vi "PSA-Mask.vi"(6 "Freq(GHZ)":dbl=20.0, 7 "Mask Offset dB":dbl, 9 "Error (dBin)":dbl, 11 "Att":dbl=0.5) -> (2 "Array":dbl[](array[numeric])=[0.5, 1.1724999999999999, 0.5862499999999999, -0.5862499999999999, 0.0], 3 "parsed result":string[](array[string]), 5 "Pass(t)":bool)   [LabVIEW 2018]
panel:
  out "Array(str)":string[](array[string])=["0.5", "1.172", "0.586", "-0.586", "0"]
  # "Error In,Atten(db),HSL,LSL,Error(db)-, Error(db)+, p/f"
  # "Error In, Atten(db),Error,Error(db)-, Error(db)+, p/f"
  # "https://ragesystems.sharepoint.com/:b:/r/sites/Tetra/Shared%20Documents/Design%20Docs/Data%20Sheets/Peregrine%20Step%20Atten%206b%2031db%2045G%20PE43614ds.pdf?csf=1&web=1&e=NTfwej"
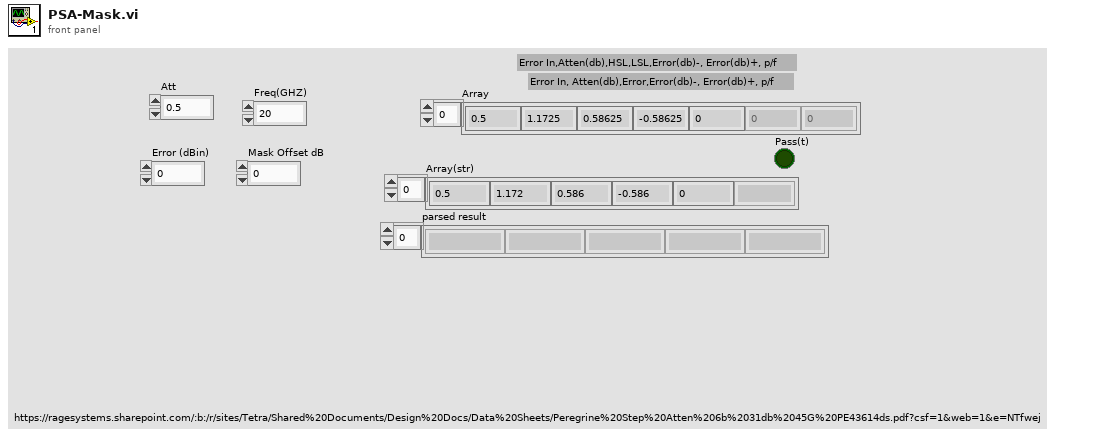
[diagram p1: front panel]
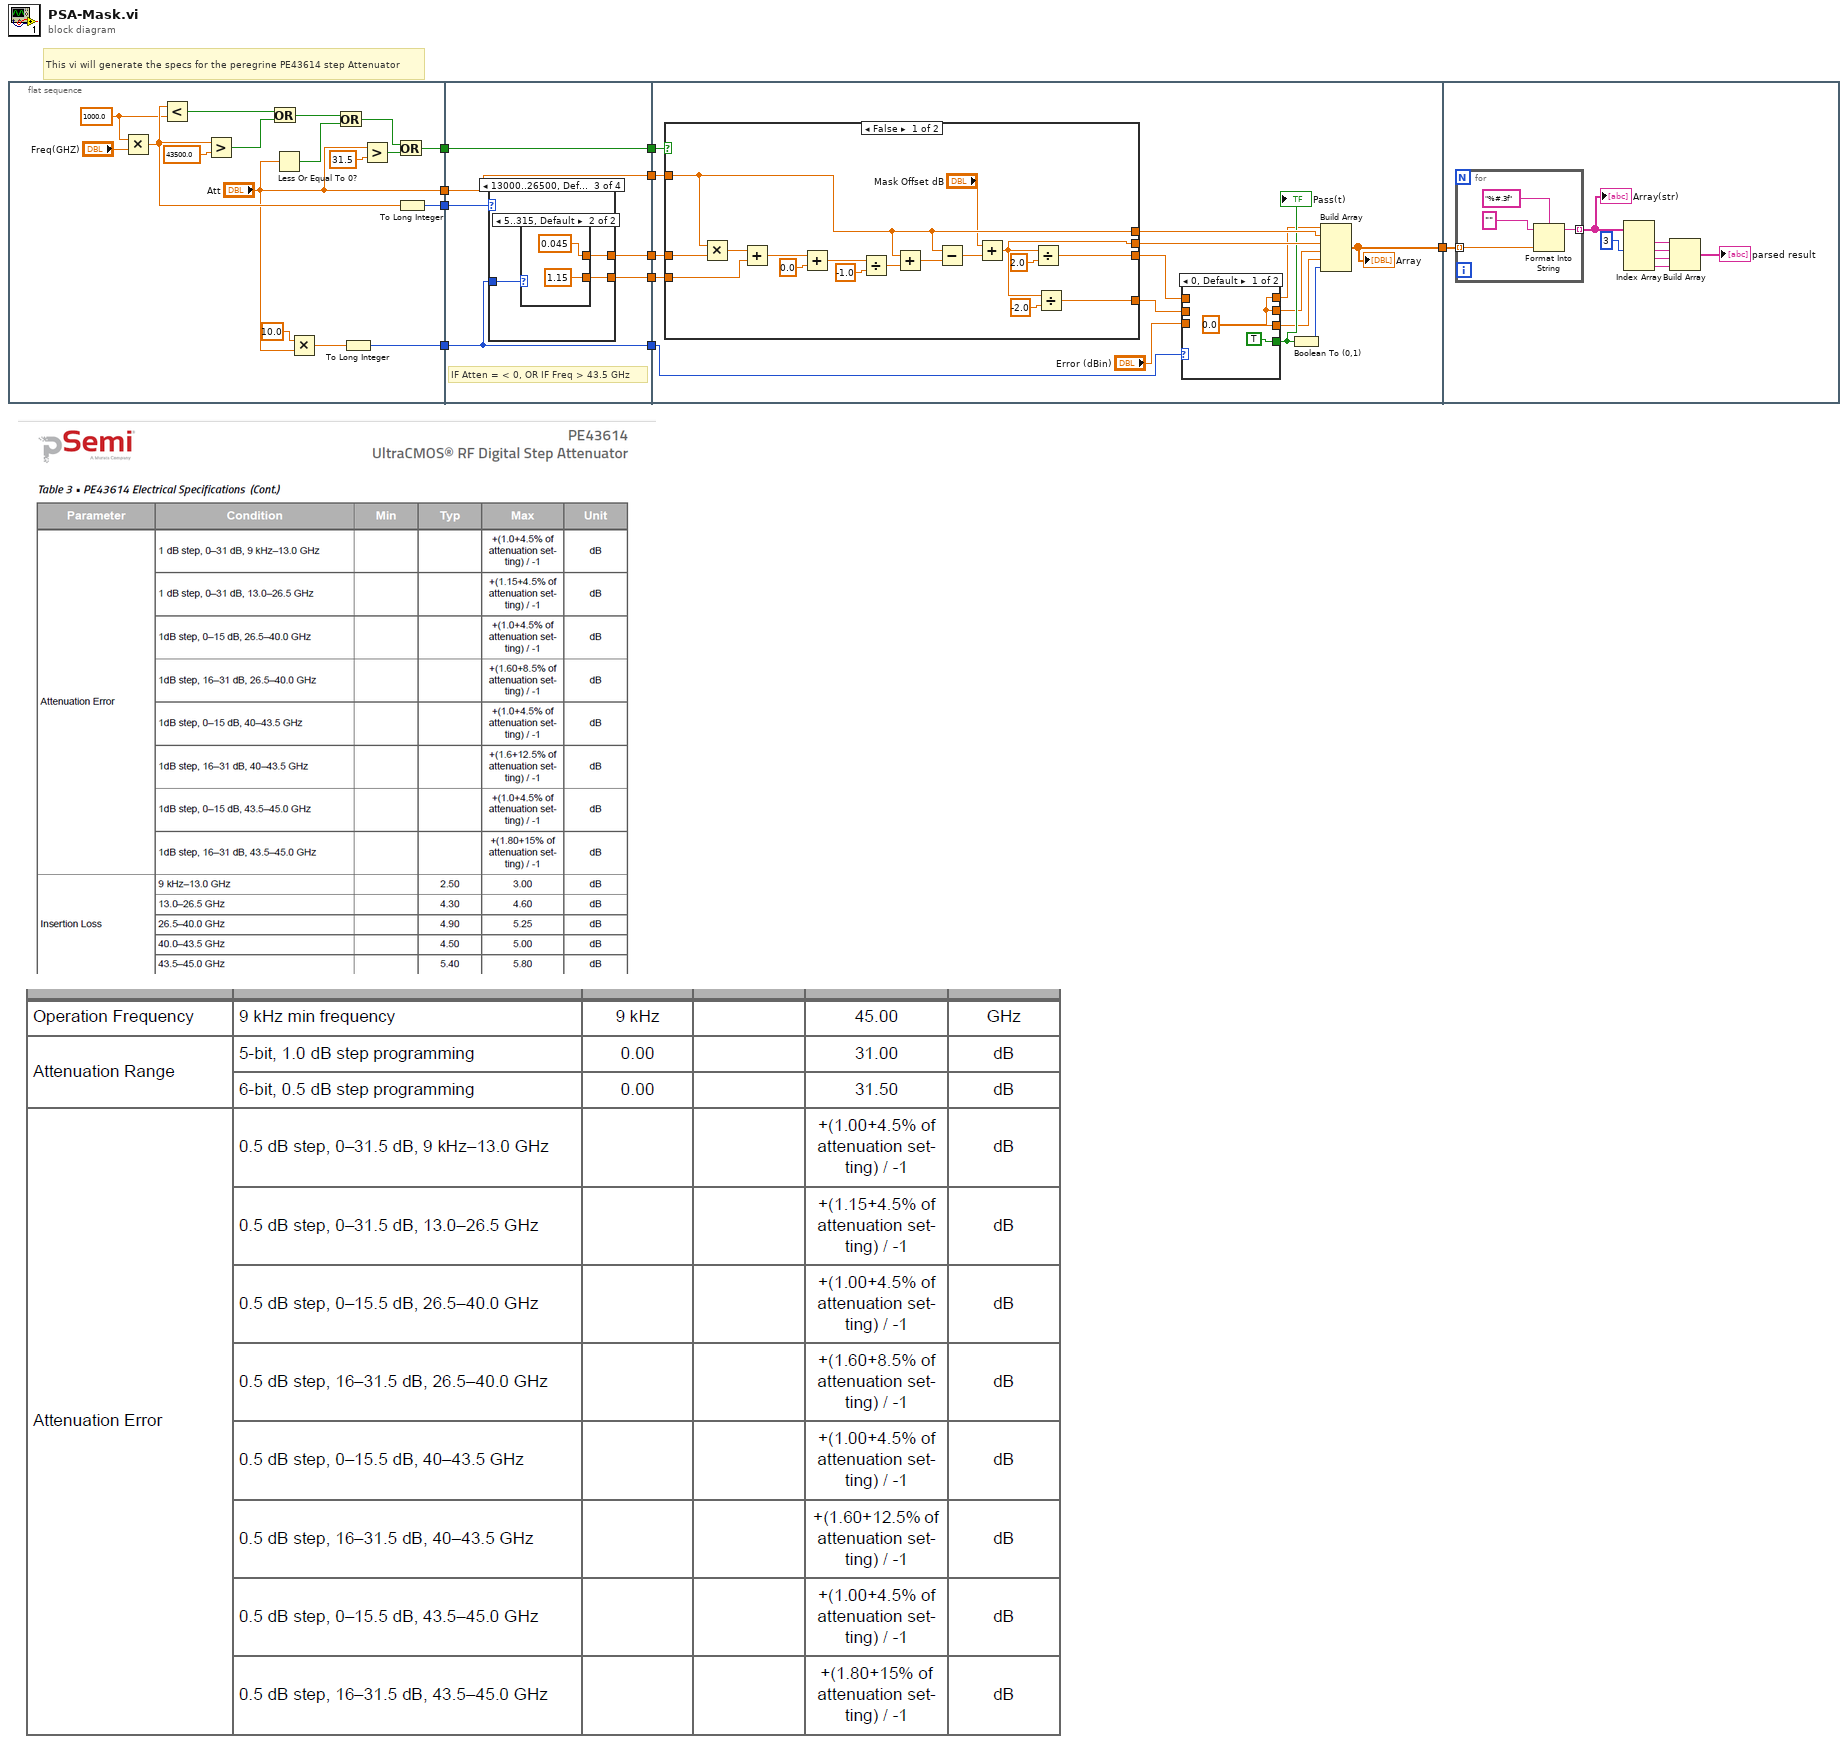
[diagram p0: block diagram]
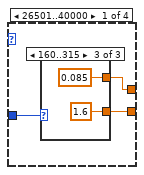
[diagram p2: hidden frame]
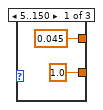
[diagram p3: hidden frame]
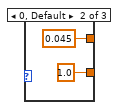
[diagram p4: hidden frame]
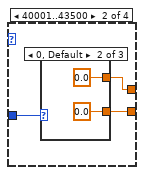
[diagram p5: hidden frame]
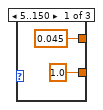
[diagram p6: hidden frame]
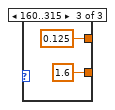
[diagram p7: hidden frame]
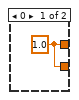
[diagram p8: hidden frame]
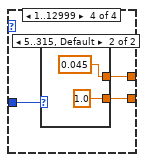
[diagram p9: hidden frame]
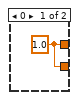
[diagram p10: hidden frame]
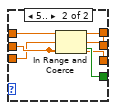
[diagram p11: hidden frame]
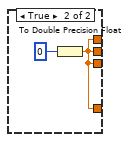
[diagram p12: hidden frame]
diagram:
  # "This vi will generate the specs for the peregrine PE43614 step Attenuator"
  n1 = flat-sequence {
    tunnel: [w25] -> w10
    tunnel: [w15] -> w9
    tunnel: [w14] -> w8
    tunnel: ["Att"] -> w7
    tunnel: w10 -> [w28]
    tunnel: w9 -> [w33]
    tunnel: w8 -> [w31]
    tunnel: w7 -> [w32]
    tunnel: [w33] -> w6
    tunnel: [w32] -> w5
    tunnel: [w30] -> w4
    tunnel: [w29] -> w3
    tunnel: [w28] -> w1
    tunnel: w6 -> [w79]
    tunnel: w5 -> [w77]
    tunnel: w4 -> [w78]
    tunnel: w3 -> [w76]
    tunnel: [w75] -> w2
    tunnel: w1 -> [w68]
    tunnel: w2 -> [w112]
    frame #0 {
      w21 = 1000.0 ("x")
      n2 = Multiply(x=w21, y="Freq(GHZ)") -> (x*y=w22:dbl)
      n3 = Less?(x=w22, y=w21) -> (x < y?=w20:bool)
      n4 = Greater?(x=w22, y=43500.0) -> (0:w19:bool)
      n5 = Or(x=w20, y=w19) -> (x .or. y?=w18:bool)
      n6 = Less Or Equal To 0?(x="Att") -> (x <= 0?=w17:bool)
      n7 = Multiply(x=10.0, y="Att") -> (x*y=w26:dbl)
      n8 = Or(x=w18, y=w17) -> (x .or. y?=w16:bool)
      n9 = To Long Integer(number=w26) -> (32bit integer=w25:i32)
      n10 = Greater?(x="Att", y=31.5) -> (0:w13:bool)
      n11 = Or(x=w16, y=w13) -> (x .or. y?=w15:bool)
      n12 = To Long Integer(number=w22) -> (32bit integer=w14:i32)
    }
    frame #1 {
      # "IF Atten = < 0, OR IF Freq > 43.5 GHz"
      n13 = case shown="13000..26500, Default" w31 {
        tunnel: [w36 w45 w54 w60] -> w30
        tunnel: [w35 w44 w53 w59] -> w29
        tunnel: w28 -> [w34 w43 w52 w58]
        frame 26501..40000 {
          n14 = case shown="160..315" w34 {
            tunnel: [0.045 ("y") 0.045 ("y") 0.085 ("y")] -> w36
            tunnel: [1.0 ("y") 1.0 ("y") 1.6 ("y")] -> w35
            frame 5..150 {
            }
            frame 0, Default {
            }
            frame 160..315 {
            }
          }
        }
        frame 40001..43500 {
          n15 = case shown="0, Default" w43 {
            tunnel: [0.045 ("y") 0.0 ("y") 0.125 ("y")] -> w45
            tunnel: [1.0 ("y") 0.0 ("y") 1.6 ("y")] -> w44
            frame 5..150 {
            }
            frame 0, Default {
            }
            frame 160..315 {
            }
          }
        }
        frame 13000..26500, Default {
          n16 = case shown="5..315, Default" w52 {
            tunnel: [w55 0.045 ("y")] -> w54
            tunnel: [w55 1.15 ("y")] -> w53
            frame 0 {
              w55 = 1.0 ("y")
            }
            frame 5..315, Default {
            }
          }
        }
        frame 1..12999 {
          n17 = case shown="5..315, Default" w58 {
            tunnel: [w61 0.045 ("y")] -> w60
            tunnel: [w61 1.0 ("y")] -> w59
            frame 0 {
              w61 = 1.0 ("y")
            }
            frame 5..315, Default {
            }
          }
        }
      }
    }
    frame #2 {
      n18 = case shown="False" w79 {
        tunnel: w78 -> [w102 _]
        tunnel: w76 -> [w101 _]
        tunnel: [w94 w103] -> w74
        tunnel: w77 -> [w94 _]
        tunnel: [w87 w103] -> w73
        tunnel: [w91 w103] -> w71
        tunnel: [w90 w103] -> w72
        frame False {
          n19 = Multiply(x=w94, y=w102) -> (x*y=w100:dbl)
          n20 = Add(x=w100, y=w101) -> (x+y=w98:dbl)
          n21 = Add(x=w98, y=0.0) -> (x+y=w97:dbl)
          n22 = Divide(x=w97, y=-1.0) -> (x/y=w95:dbl)
          n23 = Add(x=w94, y=w95) -> (x+y=w93:dbl)
          n24 = Subtract(x=w94, y=w93) -> (x-y=w86:dbl)
          n25 = Add(x="Mask Offset dB", y=w86) -> (x+y=w87:dbl)
          n26 = Divide(x=w87, y=2.0) -> (x/y=w91:dbl)
          n27 = Divide(x=w87, y=-2.0) -> (x/y=w90:dbl)
        }
        frame True {
          n28 = To Double Precision Float(number=0) -> (double precision float=w103:dbl)
        }
      }
      n29 = case shown="0, Default" w68 {
        tunnel: "Error (dBin)" -> [_ w82]
        tunnel: w72 -> [_ w83]
        tunnel: w71 -> [_ w84]
        tunnel: [TRUE w85] -> w70
        tunnel: [w80 w84] -> w66
        tunnel: [w80 w83] -> w65
        tunnel: [w80 w82] -> w64
        frame 0, Default {
          w80 = 0.0
        }
        frame 5.. {
          n30 = In Range and Coerce(upper limit=w84, x=w82, lower limit=w83) -> (In Range?=w85:bool)  [unwired: 1 out]
        }
      }
      "Pass(t)" <- w70
      n31 = Boolean To (0,1)(Boolean=w70) -> (0, 1=w69:i16)
      n32 = Build Array(w64, w74, w73, w66, w65, w69) -> (w75:dbl[])
      "Array" <- w75
    }
    frame #3 {
      n33 = for {
        tunnel: w112 -> [w116] mode=indexing
        tunnel: [w114] -> w111 mode=indexing
        n34 = Format Into String(format string="%#.3f", initial string="", w116) -> (resulting string=w114:string)  [unwired: 1 in, 1 out]
      }
      "Array(str)" <- w111
      n35 = Index Array(array=w111, index #2=3 ("index")) -> (element #1=w110:string, element #2=w109:string, element #3=w107:string, element #4=w106:string)  [unwired: 3 in]
      n36 = Build Array(w110, w109, w107, w106) -> (→"parsed result":string[])
    }
  }
